vi "Initialise Satellites.vi"(8 "error in (no error)":errorcluster, 10 "Renderer":u32, 11 "Chmmr in":refnum<class "Chmmr.lvclass">) -> (0 "error out":errorcluster, 3 "Chmmr out":refnum<class "Chmmr.lvclass">)   [LabVIEW 2021, in "Chmmr.lvclass"]
uses:
  Chmmr.lvclass
  Chmmr.lvclass/Chmmr.ctl
  Ship/Ship.lvclass
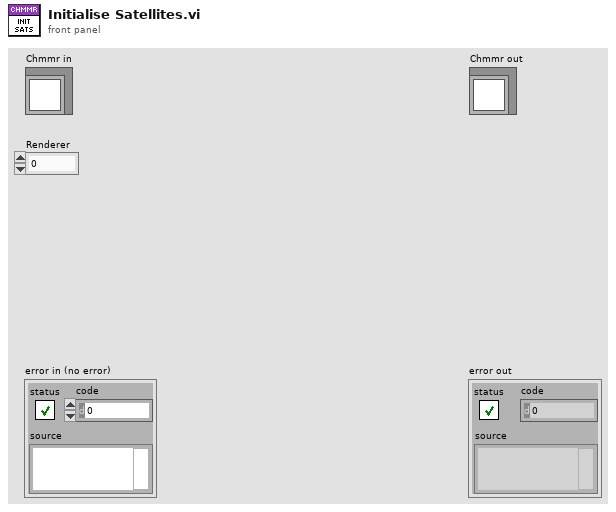
[diagram p1: front panel]
types:
  T1 = typedef "Ship.lvclass/Config.ctl" = cluster{"Race":string, "Ship Name":string, "Max Crew":i32, "Max Energy":i32, "Energy Regeneration":i32, "Weapon Energy Cost":i32, "Special Energy Cost":i32, "Energy Wait":i32, "Max Thrust":i32, "Thrust Increment":i32, "Turn Wait":i32, "Thrust Wait":i32, "Weapon Wait":i32, "Special Wait":i32, "Ship Mass":i32}
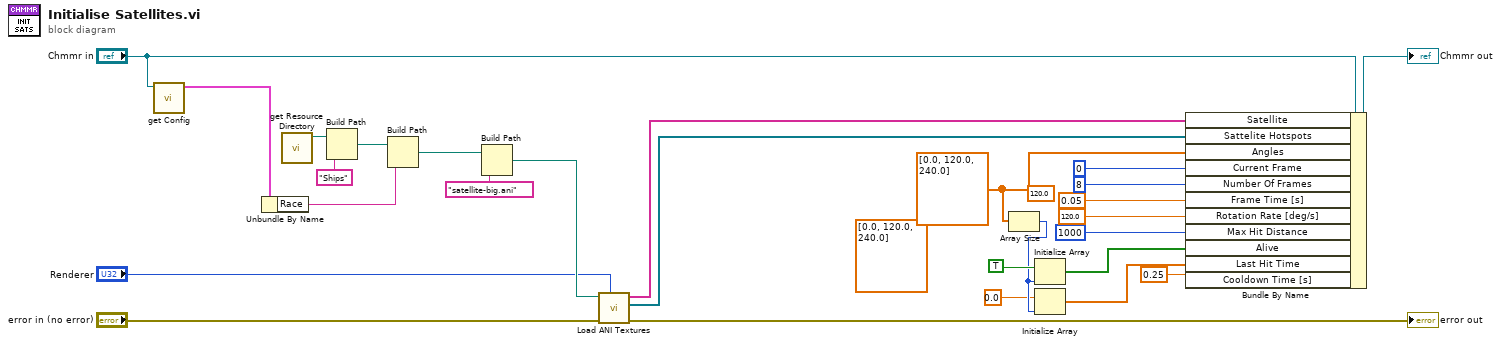
[diagram p0: block diagram]
diagram:
  (unwired) sgl[] [0.0, 120.0, 240.0] ("Satellites.Angles")
  (unwired) sgl 120.0 ("Satellites.Rotation Rate [deg/s]")
  w10 = sgl[] [0.0, 120.0, 240.0] ("Satellites.Angles")
  n1 = call "get Config.vi"("Ship in"="Chmmr in") -> ("Common"=w23:T1)  [unwired: 10 in]
  n2 = Unbundle By Name(w23) -> ("Race"=w27:string)
  n3 = call "get Resource Directory.vi"() -> ("Resource Directory"=w24:path)  [unwired: 11 in]
  n4 = Build Path(base path=w24, name or relative path="Ships") -> (appended path=w26:path)
  n5 = Build Path(base path=w26, name or relative path=w27) -> (appended path=w4:path)
  n6 = Build Path(base path=w4, name or relative path="satellite-big.ani" ("format string")) -> (appended path=w21:path)
  n7 = call "Load ANI Textures.vi"("Renderer"="Renderer", "error in (no error)"="error in (no error)", "Path"=w21) -> ("error out"=→"error out":errorcluster, "Hotspots"=w2:refnum<class "Vector 2D.lvclass">[], "Names"=w17:string[])  [unwired: 6 in]
  n8 = Array Size(array=w10) -> (size(s)=w8:i32)
  n9 = Initialize Array(TRUE, w8) -> (w9:bool[])
  n10 = Initialize Array(0.0, w8) -> (w6:dbl[])
  n11 = Bundle By Name(cluster="Chmmr in", "Satellite"=w17, "Sattelite Hotspots"=w2, "Angles"=w10, "Current Frame"=0 ("Satellites.Current Frame"), "Number Of Frames"=8 ("Satellites.Number Of Frames"), "Frame Time [s]"=0.05 ("Satellites.Frame Time [s]"), "Rotation Rate [deg/s]"=sgl 120.0 ("Satellites.Rotation Rate [deg/s]"), "Max Hit Distance"=1000 ("Satellites.Max Hit Distance"), "Alive"=w9, "Last Hit Time"=w6, "Cooldown Time [s]"=0.25) -> (→"Chmmr out":refnum<class "Chmmr.lvclass">)
